vi "sendSetServoDefaultPositionArduino.vi"(1 "servo position":u16(knob)=260 min=260 max=1150 step=1 scale=260.0..1150.0, 2 "channel":u8 max=15 step=1) -> ()   [LabVIEW 2012]
uses:
  GlobalArduino.vi
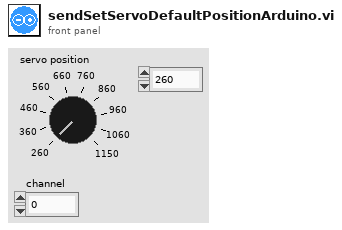
[diagram p1: front panel]
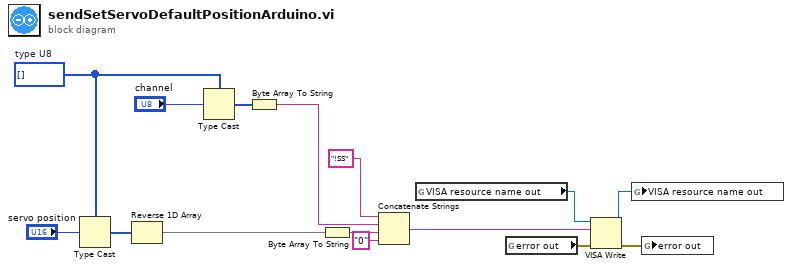
[diagram p0: block diagram]
diagram:
  w9 = u8[] []  # type U8
  n1 = Type Cast(type=w9, x="servo position") -> (*(type *) &x=w13:u8[])
  n2 = Reverse 1D Array(array=w13) -> (reversed array=w8:u8[])
  n3 = Type Cast(type=w9, x="channel") -> (*(type *) &x=w11:u8[])
  n4 = Byte Array To String(unsigned byte array=w11) -> (string=w12:string)
  n5 = Byte Array To String(unsigned byte array=w8) -> (string=w6:string)
  n6 = Concatenate Strings("!SS" ("string"), w12, w6, "0" ("string")) -> (w7:string)
  n7 = global read "GlobalArduino.vi" "VISA resource name out"() -> (w2:refnum<visa-resource-name>)
  n8 = global read "GlobalArduino.vi" "error out"() -> (w1:errorcluster)
  n9 = VISA Write(VISA resource name=w2, write buffer=w7, error in (no error)=w1) -> (VISA resource name out=w4:refnum<visa-resource-name>, error out=w3:errorcluster)  [unwired: 1 out]
  n10 = global write "GlobalArduino.vi" "VISA resource name out"(w4) -> ()
  n11 = global write "GlobalArduino.vi" "error out"(w3) -> ()
